vi "full_restart_acquire_sequence.vi"(8 "error in":errorcluster, 11 "Queue in":refnum<queue>) -> (0 "error out":errorcluster, 3 "queue out":refnum<queue>)   [LabVIEW 2012]
uses:
  typedefs/MicroscopeEvent.ctl
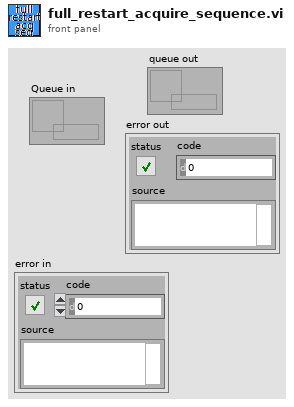
[diagram p1: front panel]
types:
  T1 = typedef "MicroscopeEvent.ctl" = enum16{"M.Wait", "M.RunRotation", "M.Flush", "M.Init", "M.InitStage", "M.InitImageData", "M.ReinitImageData", "M.ReinitImageParams", "M.GetSetParams", "M.InitFastHardware", "M.Pre-Acquire", "M.Acquire", "M.PostAcquire", "M.StopAcquire", "M.SetAcqStatusTrue", "M.SetAcqStatusFalse", "M.ClearImageData", "M.MoveStageDiscrete", "M.MoveStageToTarget1", "M.MoveStageToTarget2", "M.MoveStageToTarget3", "M.OpenShutters", "M.CloseShutters", "M.StartAcquireSequence", "M.ChangeParameters", "M.OpenStokes", "M.OpenPump", "M.RunSW"}
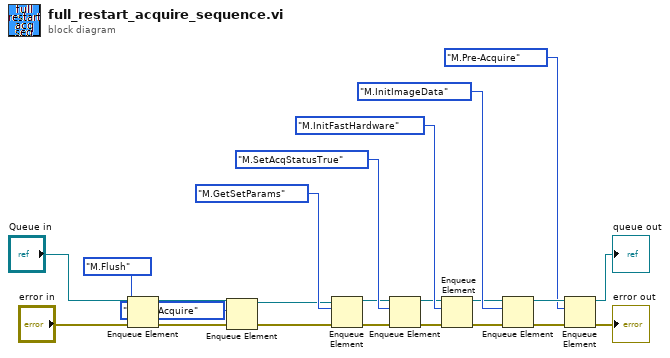
[diagram p0: block diagram]
diagram:
  n1 = Enqueue Element(queue="Queue in", element=MicroscopeEvent."M.Flush", error in (no error)="error in") -> (queue out=w3:refnum<queue>, error out=w4:errorcluster)  [unwired: 1 in, 1 out]
  n2 = Enqueue Element(queue=w3, element=MicroscopeEvent."M.PostAcquire") -> (queue out=w1:refnum<queue>)  [unwired: 2 in, 2 out]
  n3 = Enqueue Element(queue=w1, element=MicroscopeEvent."M.GetSetParams", error in (no error)=w4) -> (queue out=w8:refnum<queue>, error out=w13:errorcluster)  [unwired: 1 in, 1 out]
  n4 = Enqueue Element(queue=w8, element=MicroscopeEvent."M.SetAcqStatusTrue", error in (no error)=w13) -> (queue out=w11:refnum<queue>, error out=w12:errorcluster)  [unwired: 1 in, 1 out]
  n5 = Enqueue Element(queue=w11, element=MicroscopeEvent."M.InitFastHardware", error in (no error)=w12) -> (queue out=w17:refnum<queue>, error out=w18:errorcluster)  [unwired: 1 in, 1 out]
  n6 = Enqueue Element(queue=w17, element=MicroscopeEvent."M.InitImageData", error in (no error)=w18) -> (queue out=w21:refnum<queue>, error out=w22:errorcluster)  [unwired: 1 in, 1 out]
  n7 = Enqueue Element(queue=w21, element=MicroscopeEvent."M.Pre-Acquire", error in (no error)=w22) -> (queue out=→"queue out":refnum<queue>, error out=→"error out":errorcluster)  [unwired: 1 in, 1 out]
